vi "ComVenus.vi"() -> ()   [LabVIEW 2017]
panel:
  out "lat_mercury 2":dbl
  out "lat_mercury":dbl
  in  "stop":bool
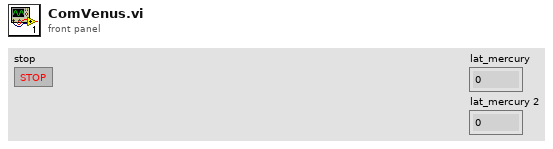
[diagram p1: front panel]
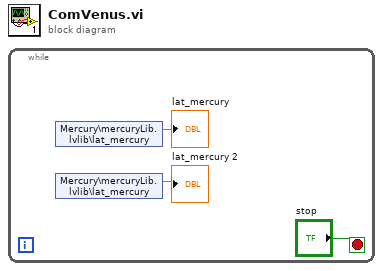
[diagram p0: block diagram]
diagram:
  n1 = while {
    stop <- "stop" stop-if-true
    n2 = shared-variable "Mercury\\mercuryLib.lvlib\\lat_mercury"() -> (→"lat_mercury":dbl)  [unwired: 1 in, 1 out]
    n3 = shared-variable "Mercury\\mercuryLib.lvlib\\lat_mercury"() -> (→"lat_mercury 2":dbl)  [unwired: 1 in, 1 out]
  }
